vi "DataListenerRepository.vi"(0 "Connection ID":u64, 1 "Action(ReadRepository)":T1(ring), 5 "error in (no error)":errorcluster) -> (9 "ProcessViRef":refnum<vi>, 11 "ProcessSyncQueue":refnum<queue>, 13 "FromProcessQueue":refnum<queue>, 15 "ToProcessQueue":refnum<queue>, 17 "ProcessAlreadyStarted":bool, 19 "error out":errorcluster)   [LabVIEW 2014, in "FrontPanelPublisher.lvlib" / "Websocket.lvclass"]
uses:
  Websocket.lvclass
  DataListener.ctl
  DataListener.vi
panel:
  # "Use this indicator for sending messages to the Process VI"
  # "These indicators are used by the process VIs"
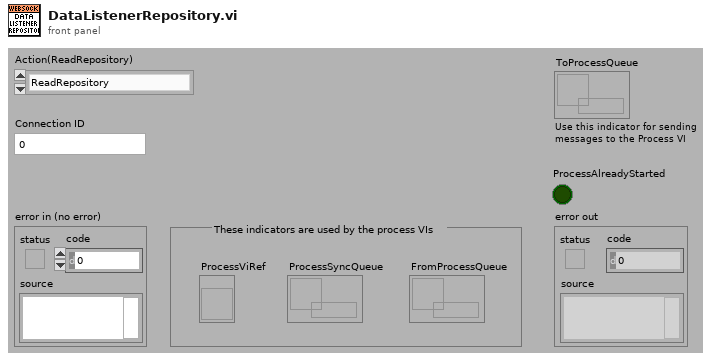
[diagram p1: front panel]
types:
  T1 = enum16{"ReadRepository", "CreateNew", "CreateOrLookUpExisting", "ReadRepositoryAndDestroy"}
  T2 = typedef "FrontPanelPublisher.lvlib/Websocket.lvclass/DataListener.ctl" = cluster{"ToProcessQueue":refnum<queue>, "FromProcessQueue":refnum<queue>, "ProcessSyncQueue":refnum<queue>, "ProcessViRef":refnum<vi>}
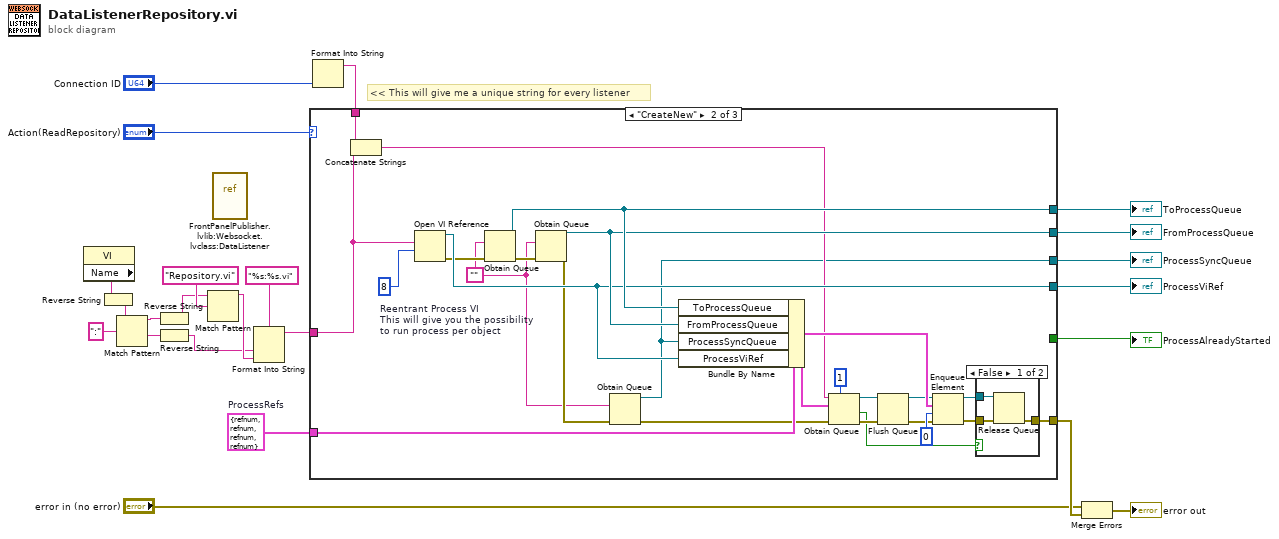
[diagram p0: block diagram]
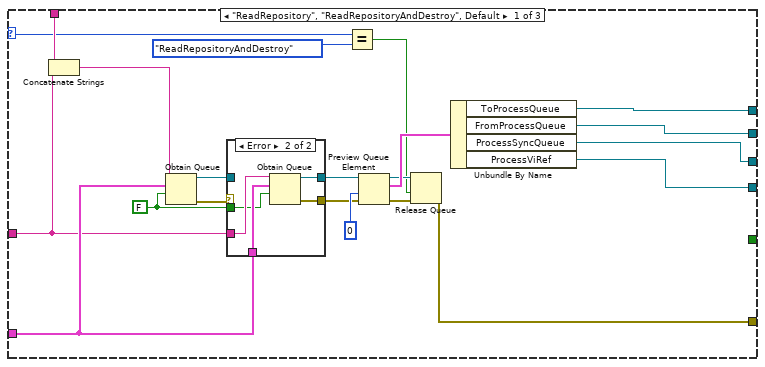
[diagram p2: hidden frame]
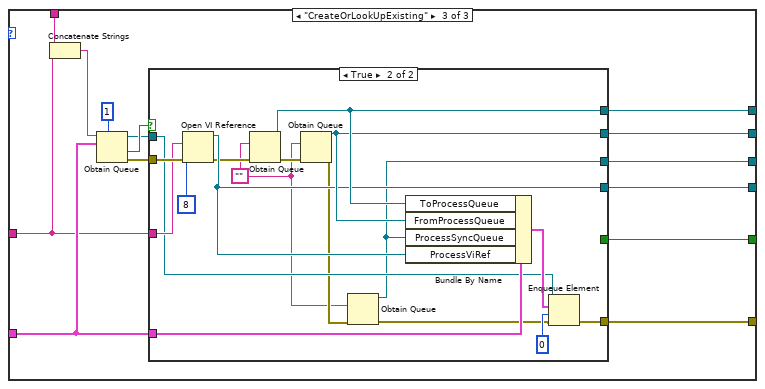
[diagram p5: hidden frame]
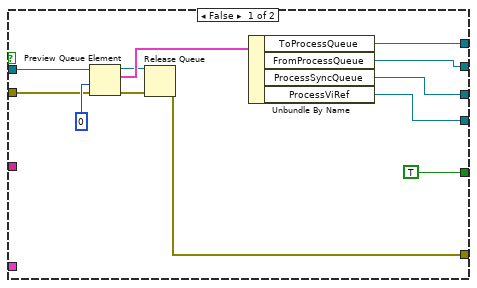
[diagram p6: hidden frame]
diagram:
  w18 = T2 {"ToProcessQueue"=refnum, "FromProcessQueue"=refnum, "ProcessSyncQueue"=refnum, "ProcessViRef"=refnum}  # ProcessRefs
  # "<< This will give me a unique string for every listener"
  n1 = property class="VI"() -> ("Name"=w7:string)  [unwired: 2 in, 2 out]
  n2 = Reverse String(1:w7) -> (0:w8:string)
  n3 = Match Pattern(string=w8, regular expression=":") -> (before substring=w12:string, after substring=w9:string)  [unwired: 1 in, 2 out]
  n4 = Reverse String(1:w12) -> (0:w13:string)
  n5 = Reverse String(1:w9) -> (0:w11:string)
  n6 = Match Pattern(string=w13, regular expression="Repository.vi") -> (before substring=w15:string)  [unwired: 1 in, 3 out]
  n7 = vi-ref "FrontPanelPublisher.lvlib:Websocket.lvclass:DataListener.vi"() -> ()  [unwired: 1 out]
  n8 = Format Into String(format string="%s:%s.vi", w11, w15) -> (resulting string=w5:string)  [unwired: 2 in, 1 out]
  n9 = Format Into String("Connection ID") -> (resulting string=w2:string)  [unwired: 3 in, 1 out]
  n10 = case shown="\"CreateNew\"" "Action(ReadRepository)" {
    selector: "Action(ReadRepository)" -> [w25 _ _]
    tunnel: [w39 w60 w92] -> w22
    tunnel: [w41 w76 w94] -> w20
    tunnel: [w40 w75 w93] -> w21
    tunnel: [w42 w74 w91] -> w19
    tunnel: w18 -> [w34 w66 w87]
    tunnel: w2 -> [w32 w65 w83]
    tunnel: [w27 w54 w90] -> w16
    tunnel: w5 -> [w31 w63 w82]
    tunnel: [_ _ w85] -> w4
    frame "ReadRepository", "ReadRepositoryAndDestroy", Default {
      w33 = FALSE ("create if not found? (T)")
      n11 = Concatenate Strings(w32, w31) -> (w30:string)
      n12 = Obtain Queue(name (unnamed)=w30, element data type=w34, create if not found? (T)=w33) -> (queue out=w36:refnum<queue>, error out=w38:errorcluster)  [unwired: 2 in, 1 out]
      n13 = case shown="Error" w38 {
        selector: w38 -> [w46 _]
        tunnel: [w46 w48] -> w37
        tunnel: w36 -> [w45 _]
        tunnel: [w45 w49] -> w35
        tunnel: w34 -> [_ w51]
        tunnel: w31 -> [_ w50]
        tunnel: w33 -> [_ w47]
        frame No Error {
        }
        frame Error {
          n14 = Obtain Queue(name (unnamed)=w50, element data type=w51, create if not found? (T)=w47) -> (queue out=w49:refnum<queue>, error out=w48:errorcluster)  [unwired: 2 in, 1 out]
        }
      }
      n15 = Equal?(x=w25, y=T1."ReadRepositoryAndDestroy") -> (x = y?=w24:bool)
      n16 = Preview Queue Element(queue=w35, timeout in ms (-1)=0, error in (no error)=w37) -> (queue out=w29:refnum<queue>, element=w43:T2, error out=w28:errorcluster)  [unwired: 1 out]
      n17 = Release Queue(queue=w29, force destroy? (F)=w24, error in (no error)=w28) -> (error out=w27:errorcluster)  [unwired: 2 out]
      n18 = Unbundle By Name(w43) -> ("ToProcessQueue"=w41:refnum<queue>, "FromProcessQueue"=w40:refnum<queue>, "ProcessSyncQueue"=w39:refnum<queue>, "ProcessViRef"=w42:refnum<vi>)
    }
    frame "CreateNew" {
      w71 = 8  # Reentrant Process VI This will give you the possibility to run process per object
      w52 = ""
      n19 = Concatenate Strings(w65, w63) -> (w64:string)
      n20 = Open VI Reference(vi path=w63, options=w71) -> (vi reference=w74:refnum<vi>, error out=w72:errorcluster)  [unwired: 4 in]
      n21 = Obtain Queue(element data type=w52, error in (no error)=w72) -> (queue out=w76:refnum<queue>, error out=w73:errorcluster)  [unwired: 3 in, 1 out]
      n22 = Obtain Queue(element data type=w52, error in (no error)=w73) -> (queue out=w75:refnum<queue>, error out=w62:errorcluster)  [unwired: 3 in, 1 out]
      n23 = Obtain Queue(element data type=w52, error in (no error)=w62) -> (queue out=w60:refnum<queue>, error out=w61:errorcluster)  [unwired: 3 in, 1 out]
      n24 = Bundle By Name(cluster=w66, "ToProcessQueue"=w76, "FromProcessQueue"=w75, "ProcessSyncQueue"=w60, "ProcessViRef"=w74) -> (w69:T2)
      n25 = Obtain Queue(max queue size (-1, unlimited)=1, name (unnamed)=w64, element data type=w69, error in (no error)=w61) -> (queue out=w70:refnum<queue>, created new?=w53:bool, error out=w58:errorcluster)  [unwired: 1 in]
      n26 = Flush Queue(queue=w70, error in (no error)=w58) -> (queue out=w59:refnum<queue>, error out=w57:errorcluster)  [unwired: 1 out]
      n27 = Enqueue Element(queue=w59, element=w69, timeout in ms (-1)=0, error in (no error)=w57) -> (queue out=w56:refnum<queue>, error out=w55:errorcluster)  [unwired: 1 out]
      n28 = case shown="False" w53 {
        tunnel: w55 -> [w79 w80]
        tunnel: w56 -> [w78 _]
        tunnel: [w77 w80] -> w54
        frame False {
          n29 = Release Queue(queue=w78, error in (no error)=w79) -> (error out=w77:errorcluster)  [unwired: 1 in, 2 out]
        }
        frame True {
        }
      }
    }
    frame "CreateOrLookUpExisting" {
      n30 = Concatenate Strings(w83, w82) -> (w81:string)
      n31 = Obtain Queue(max queue size (-1, unlimited)=1, name (unnamed)=w81, element data type=w87) -> (queue out=w88:refnum<queue>, created new?=w89:bool, error out=w86:errorcluster)  [unwired: 2 in]
      n32 = case shown="True" w89 {
        tunnel: [w106 w123] -> w94
        tunnel: [w105 w122] -> w93
        tunnel: [w104 w109] -> w92
        tunnel: [w103 w121] -> w91
        tunnel: [w95 w120] -> w90
        tunnel: w87 -> [_ w119]
        tunnel: w86 -> [w100 w114]
        tunnel: w82 -> [_ w113]
        tunnel: w88 -> [w101 w112]
        tunnel: [TRUE _] -> w85
        frame False {
          n33 = Preview Queue Element(queue=w101, timeout in ms (-1)=0, error in (no error)=w100) -> (queue out=w97:refnum<queue>, element=w99:T2, error out=w96:errorcluster)  [unwired: 1 out]
          n34 = Release Queue(queue=w97, error in (no error)=w96) -> (error out=w95:errorcluster)  [unwired: 1 in, 2 out]
          n35 = Unbundle By Name(w99) -> ("ToProcessQueue"=w106:refnum<queue>, "FromProcessQueue"=w105:refnum<queue>, "ProcessSyncQueue"=w104:refnum<queue>, "ProcessViRef"=w103:refnum<vi>)
        }
        frame True {
          w108 = ""
          n36 = Open VI Reference(vi path=w113, options=8, error in (no error)=w114) -> (vi reference=w121:refnum<vi>, error out=w117:errorcluster)  [unwired: 3 in]
          n37 = Obtain Queue(element data type=w108, error in (no error)=w117) -> (queue out=w123:refnum<queue>, error out=w118:errorcluster)  [unwired: 3 in, 1 out]
          n38 = Obtain Queue(element data type=w108, error in (no error)=w118) -> (queue out=w122:refnum<queue>, error out=w111:errorcluster)  [unwired: 3 in, 1 out]
          n39 = Obtain Queue(element data type=w108, error in (no error)=w111) -> (queue out=w109:refnum<queue>, error out=w110:errorcluster)  [unwired: 3 in, 1 out]
          n40 = Bundle By Name(cluster=w119, "ToProcessQueue"=w123, "FromProcessQueue"=w122, "ProcessSyncQueue"=w109, "ProcessViRef"=w121) -> (w116:T2)
          n41 = Enqueue Element(queue=w112, element=w116, timeout in ms (-1)=0, error in (no error)=w110) -> (error out=w120:errorcluster)  [unwired: 2 out]
        }
      }
    }
  }
  "ProcessSyncQueue" <- w22
  "ToProcessQueue" <- w20
  "FromProcessQueue" <- w21
  "ProcessViRef" <- w19
  "ProcessAlreadyStarted" <- w4
  n42 = Merge Errors("error in (no error)", w16) -> (→"error out":errorcluster)
